vi "Read Pulse Data Points.vi"(8 "error in":errorcluster, 11 "Electronic Load in":refnum<class "Electronic Load.lvclass">) -> (0 "error out":errorcluster, 2 "Data Pts":i32, 3 "Electronic Load out":refnum<class "Electronic Load.lvclass">)   [LabVIEW 2019, in "Electronic Load.lvlib" / "Electronic Load.lvclass"]
uses:
  Library/Electronic Load.lvclass
  Library/Electronic Load.lvclass/Electronic Load.ctl
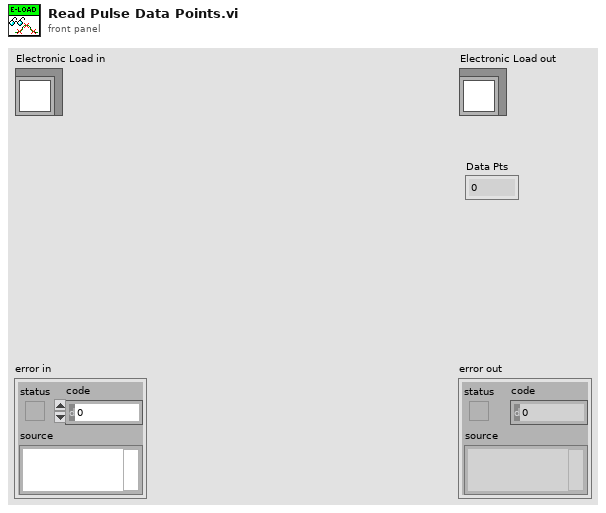
[diagram p1: front panel]
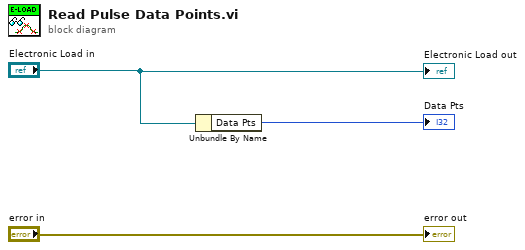
[diagram p0: block diagram]
diagram:
  n1 = Unbundle By Name("Electronic Load in") -> ("Data Pts"=→"Data Pts":i32)
  "error out" <- "error in"
  "Electronic Load out" <- "Electronic Load in"
